vi "RT_timing.vi"() -> ()   [LabVIEW 2017]
uses:
  <vilib>/Platform/TimedLoop/XDataNode/timing_clust.ctl
  <vilib>/Platform/TimedLoop/XDataNode/nitl_modes.ctl
  <vilib>/Platform/TimedLoop/XDataNode/wakeup.ctl
  <vilib>/myRIO/Instrument Drivers/Onboard Devices/Accelerometer/typedefs/Accelerometer Reference.ctl
  <vilib>/myRIO/Common/Instrument Driver Framework/Utilities/typedefs/myRIO Generic Hardware Reference.ctl
  <vilib>/myRIO/Common/Instrument Driver Framework/Utilities/typedefs/Hardware Version Enum.ctl
  <vilib>/myRIO/Common/Instrument Driver Framework/Utilities/typedefs/myRIO v1.0 Reference.ctl
  <vilib>/myRIO/Common/Instrument Driver Framework/Utilities/typedefs/Generic FPGA Reference.ctl
  <vilib>/myRIO/Common/Instrument Driver Framework/myRIO v1.0/Accelerometer/typedefs/Accelerometer Channels List.ctl
  <vilib>/myRIO/Common/Instrument Driver Framework/myRIO v1.0/Accelerometer/typedefs/Accelerometer Channels Enum.ctl
  <vilib>/userdefined/High Color/nirio_resource_hc.ctl
  <vilib>/myRIO/Instrument Drivers/Onboard Devices/Accelerometer/vis/Read.vi
  <vilib>/myRIO/Common/Instrument Driver Framework/myRIO v1.0/Accelerometer/vis/myRIO v1.1 Open Accelerometer.vi
  <vilib>/myRIO/Common/Instrument Driver Framework/Utilities/vis/Is FPGA Ref Available.vi
  <vilib>/myRIO/Common/Instrument Driver Framework/Utilities/vis/Validate Channels.vi
  <vilib>/myRIO/Common/Instrument Driver Framework/myRIO v1.0/Accelerometer/vis/myRIO v1.0 Reserve Accelerometer.vi
  <vilib>/myRIO/Common/Instrument Driver Framework/myRIO v1.0/Resource Manager/vis/myRIO v1.0 Reserve Channel List.vi
  <vilib>/myRIO/Common/Instrument Driver Framework/myRIO v1.0/Accelerometer/vis/myRIO v1.0 Build MUX Configuration Accelerometer.vi
  <vilib>/myRIO/Common/Instrument Driver Framework/myRIO v1.0/Resource Manager/vis/myRIO v1.0 Reserve Channel.vi
  <vilib>/myRIO/Common/Instrument Driver Framework/myRIO v1.0/Resource Manager/vis/myRIO v1.0 Unreserve Channel.vi
  <vilib>/myRIO/Common/Instrument Driver Framework/myRIO v1.0/Resource Manager/vis/myRIO v1.0 Build Mutex Name.vi
  <vilib>/myRIO/Common/Instrument Driver Framework/myRIO v1.0/Accelerometer/vis/myRIO v1.0 Read Accelerometer.vi
  <vilib>/Utility/error.llb/Error Cluster From Error Code.vi
  <vilib>/myRIO/Common/Instrument Driver Framework/myRIO v1.0/myRIO v1.0 Close.vi
  <vilib>/myRIO/Common/Instrument Driver Framework/Utilities/vis/IO Manager.vi
  <vilib>/myRIO/Common/Instrument Driver Framework/Utilities/vis/Configuration Manager.vi
  <vilib>/myRIO/Common/Instrument Driver Framework/myRIO v1.0/Accelerometer/vis/myRIO v1.0 Get Scaling Constant Accelerometer.vi
  <vilib>/myRIO/Common/Instrument Driver Framework/myRIO v1.0/myRIO v1.1 Open.vi
  <vilib>/Utility/VariantDataType/GetNumericInfo.vi
  <vilib>/platform/TimedLoop/XDataNode/XDataNode.xnode
  <vilib>/myRIO/Instrument Drivers/Onboard Devices/Accelerometer/vis/myRIO Accelerometer Open.xnode
  <vilib>/myRIO/Express VI/Onboard Devices/Accelerometer/Accelerometer Express VI.xnode
  <vilib>/Platform/TimedLoop/XDataNode/XDNodeRunTimeDep.lvlib
  <vilib>/myRIO/Instrument Drivers/Onboard Devices/Accelerometer/Accelerometer.lvlib
panel:
  in  "Tab Control":T1(tab)
  out "Waveform Chart":i64(graph)
  out "RT_LoopTime":u32
  out "Loop_time":i32
  out "RT_Time":u32
  out "Num_iteration":i32
  in  "stop":bool
  out "s? t:f":i64
  out "Waveform Chart 3":u32(graph)
  out "Time_Iteration 2":i32
  in  "stop 3":bool
  out "Time_RT 2":u32
  out "Time_RT":u32
  in  "stop 2":bool
  out "Time_Iteration":i32
  out "Waveform Chart 2":u32(graph)
  # "Time_unit us"
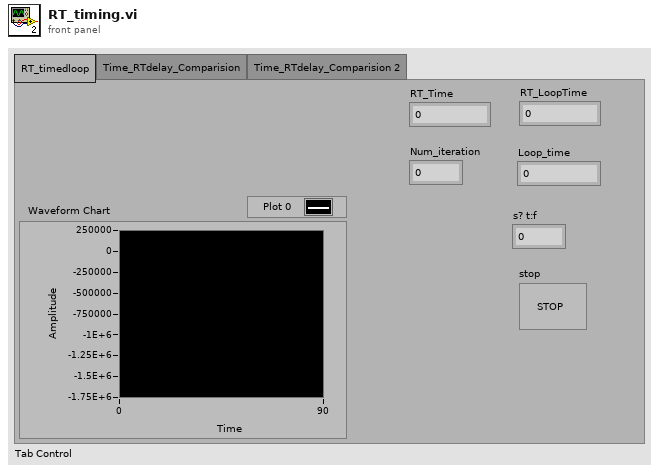
[diagram p1: front panel]
types:
  T1 = enum32{"RT_timedloop", "Time_RTdelay_Comparision", "Time_RTdelay_Comparision 2"}
  T2 = typedef "XDNodeRunTimeDep.lvlib/timing_clust.ctl" = cluster{"Expected End [f-1]":u64, "Actual End [f-1]":u64, "Finished Late? [f-1]":bool, "Expected End [i-1]":u64, "Actual End [i-1]":u64, "Finished Late? [i-1]":bool, "Expected Start [i]":u64, "Actual Start [i]":u64, "Expected Start [f]":u64, "Actual Start [f]":u64, "Source Name":string, "Structure Name":string, "Period":i64, "Deadline":i64, "Offset":i64, "Start":i64, "Priority":i32, "Timeout":i32, "Mode":T3, "Wakeup Reason":T4, "Error":errorcluster, "Source Type":string, "Secondary Source Type":string, "Global End Time":u64, "Global Start Time":u64, "Frame Duration":u64, "Iteration Duration":u64, "Assigned CPU":i32, "I/O Scan Engine Mode":u32}
  T3 = typedef "XDNodeRunTimeDep.lvlib/nitl_modes.ctl" = enum32{"No Change", "Process missed periods, maintain original phase", "Discard missed periods, maintain original phase", "Process missed periods, ignore original phase", "Discard missed periods, ignore original phase"}
  T4 = typedef "XDNodeRunTimeDep.lvlib/wakeup.ctl" = enum32{"Normal", "Aborted", "Asynchronous wakeup", "Timing source error", "Timed loop error", "Timeout"}
  T5 = typedef "Accelerometer.lvlib/Accelerometer Reference.ctl" = cluster{"myRIO Reference":T6, "Accelerometer Channels List":T10, "LSB Weight":dbl}
  T6 = typedef "myRIO Generic Hardware Reference.ctl" = cluster{"myRIO Model":T7, "myRIO Hardware Reference":T8}
  T7 = typedef "Hardware Version Enum.ctl" = enum16{"Unknown", "myRIO-1900", "myRIO-1950", "roboRIO", "NI ELVIS RIO CM"}
  T8 = typedef "myRIO v1.0 Reference.ctl" = cluster{"Generic FPGA Reference":T9, "Allow multiple opens":bool}
  T9 = typedef "Generic FPGA Reference.ctl" = refnum<k20>
  T10 = typedef "Accelerometer Channels List.ctl" = T11[]
  T11 = typedef "Accelerometer Channels Enum.ctl" = enum16{"Not Connected", "X-Axis", "Y-Axis", "Z-Axis"}
  T12 = typedef "nirio_resource_hc.ctl" = tag
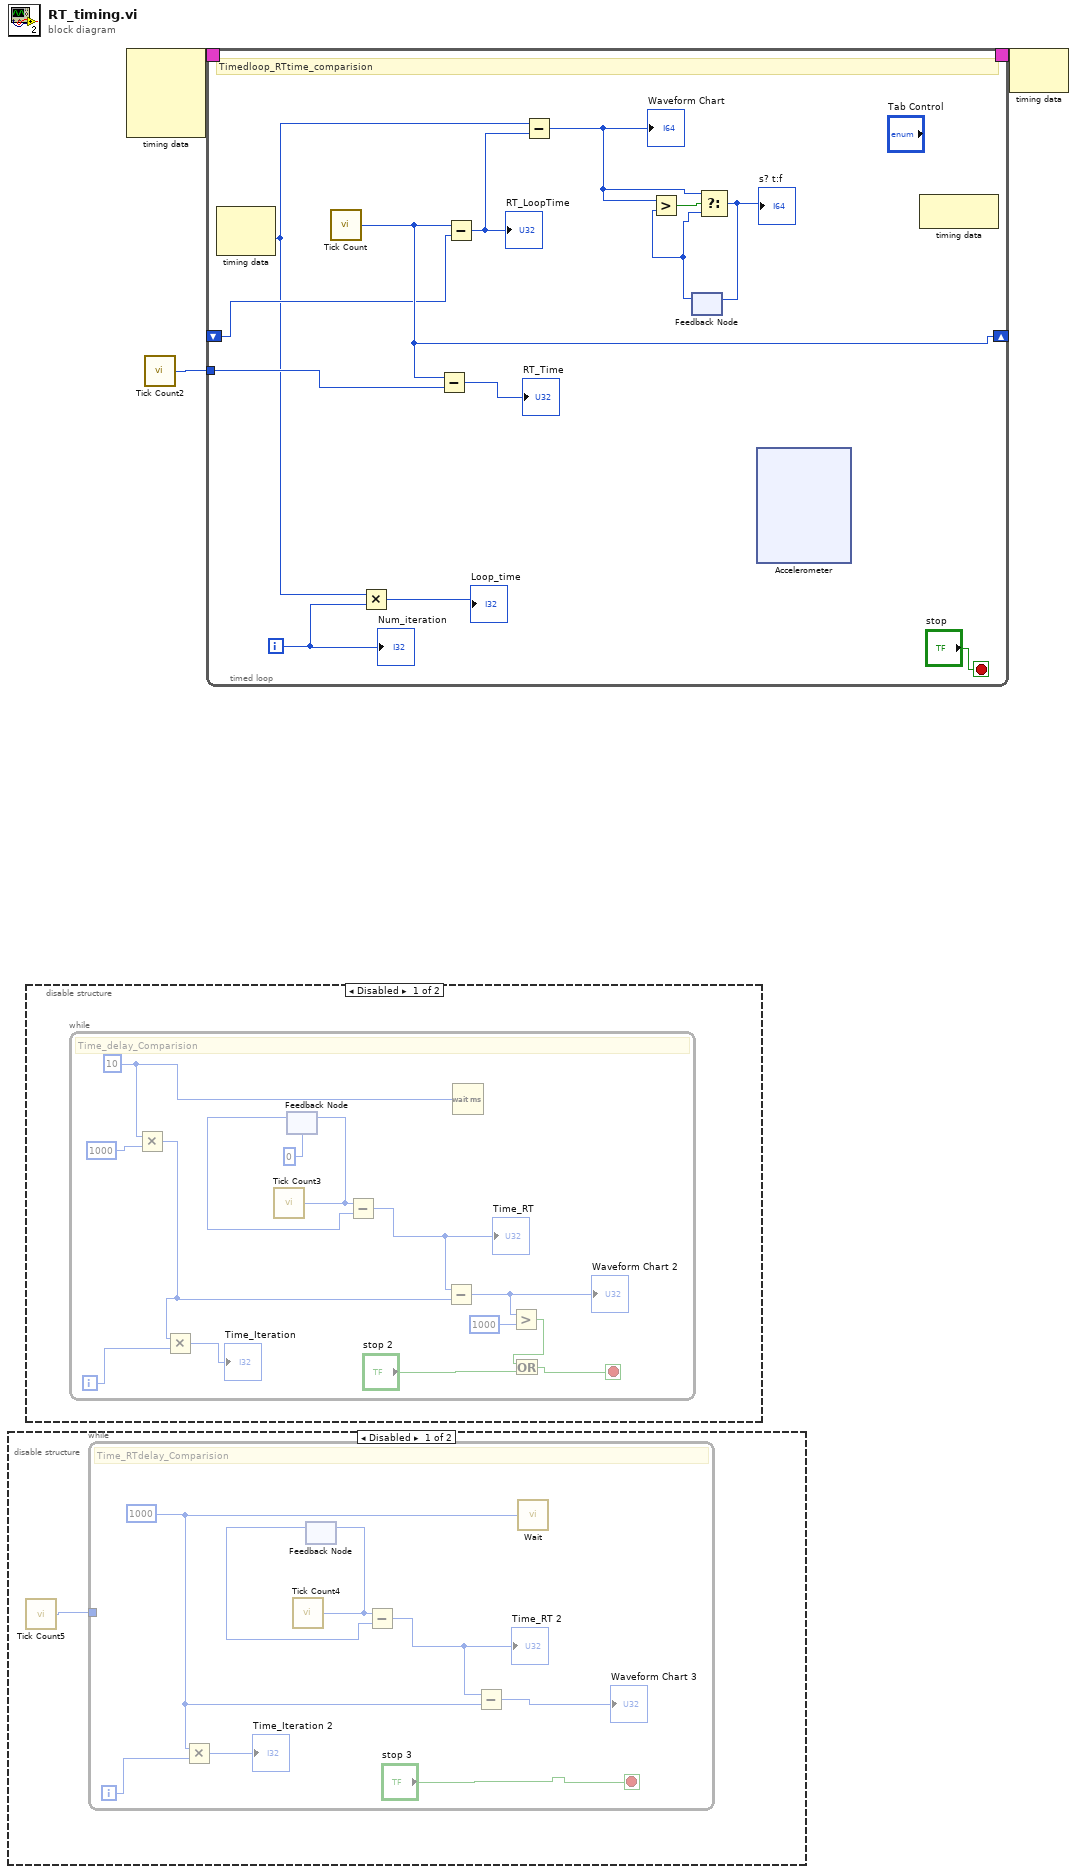
[diagram p0: block diagram]
diagram:
  n1 = disable-structure shown="Disabled" {
    frame Disabled {
      n2 = call "Tick Count5"() -> ("Tick Count(uSec)"=w4:u32)
      n3 = while {
        tunnel: w4 -> [_]
        i -> [w11]
        stop <- "stop 3" stop-if-true
        w6 = u32 1000 ("Count(uSec)")
        # "Time_RTdelay_Comparision"
        n4 = Multiply(x=w6, y=w11) -> (x*y=→"Time_Iteration 2":u32)
        n5 = call "Tick Count4"() -> ("Tick Count(uSec)"=w9:u32)
        n6 = feedback-in #1(w9) -> ()
        n7 = feedback #1() -> (w8:u32)  [unwired: 1 in]
        n8 = Subtract(x=w9, y=w8) -> (x-y=w10:u32)
        "Time_RT 2" <- w10
        n9 = Subtract(x=w10, y=w6) -> (x-y=→"Waveform Chart 3":u32)
        n10 = call "Wait"("Count(uSec)"=w6) -> ()  [unwired: 1 out]
      }
    }
    frame Enabled {
    }
  }
  n11 = disable-structure shown="Disabled" {
    frame Disabled {
      n12 = while {
        i -> [w25]
        stop <- w13 stop-if-true
        w23 = u32 10 ("Count(uSec)")
        # "Time_delay_Comparision"
        n13 = Multiply(x=w23, y=u32 1000) -> (x*y=w22:u32)
        n14 = Multiply(x=w22, y=w25) -> (x*y=→"Time_Iteration":u32)
        n15 = call "Tick Count3"() -> ("Tick Count(uSec)"=w20:u32)
        n16 = feedback-in #2(w20) -> ()
        n17 = feedback #2(u32 0 ("Tick Count(uSec)")) -> (w19:u32)
        n18 = Subtract(x=w20, y=w19) -> (x-y=w21:u32)
        "Time_RT" <- w21
        n19 = Subtract(x=w21, y=w22) -> (x-y=w16:u32)
        "Waveform Chart 2" <- w16
        n20 = Wait (ms)(milliseconds to wait=w23) -> ()  [unwired: 1 out]
        n21 = Greater?(x=w16, y=u32 1000) -> (0:w14:bool)
        n22 = Or(x=w14, y="stop 2") -> (x .or. y?=w13:bool)
      }
    }
    frame Enabled {
    }
  }
  n23 = node-c288() -> (w3:T2)  [unwired: 4 in]
  n24 = call "Tick Count2"() -> ("Tick Count(uSec)"=w1:u32)
  n25 = timed-loop {
    timing: w3 -> [_]
    timing-out: [_] -> w2
    tunnel: w1 -> [w38]
    shift-right: [w34] -> _
    shift-left: _ -> [w33]
    i -> [w36]
    stop <- "stop" stop-if-true
    # "Timedloop_RTtime_comparision"
    n26 = node-c288() -> (w31:i64)  [unwired: 1 in, 1 out]
    n27 = call "Tick Count"() -> ("Tick Count(uSec)"=w34:u32)
    n28 = Multiply(x=w31, y=w36) -> (x*y=→"Loop_time":i64)
    n29 = Subtract(x=w34, y=w38) -> (x-y=→"RT_Time":u32)
    n30 = Subtract(x=w34, y=w33) -> (x-y=w32:u32)
    "RT_LoopTime" <- w32
    n31 = Subtract(x=w31, y=w32) -> (x-y=w29:i64)
    "Waveform Chart" <- w29
    n32 = feedback #3() -> (w27:i64)  [unwired: 1 in]
    n33 = Greater?(x=w29, y=w27) -> (0:w30:bool)
    n34 = Select(t=w29, s=w30, f=w27) -> (s? t:f=w28:i64)
    "s? t:f" <- w28
    n35 = feedback-in #3(w28) -> ()
    n36 = xnode "Accelerometer"() -> ()  [unwired: 1 in, 4 out]
    n37 = node-c288() -> ()  [unwired: 1 in, 1 out]
    "Num_iteration" <- w36
  }
  n38 = node-c288(w2) -> ()  [unwired: 1 out]
